vi "Set Isolated Crop Mode.vi"(6 "hbin":i32, 7 "vbin":i32, 9 "cropwidth":i32, 10 "cropheight":i32, 11 "active":i32) -> (3 "function return":u32)   [LabVIEW 2018, in "AndorSDK.lvlib"]
doc: "EXPNETTYPE unsigned int WINAPI SetIsolatedCropMode(int active, int cropheight, int cropwidth, int vbin, int hbin);"
uses:
  AndorSDK.lvlib
  ATMCD32D.dll
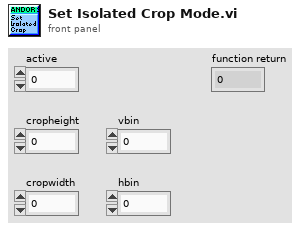
[diagram p1: front panel]
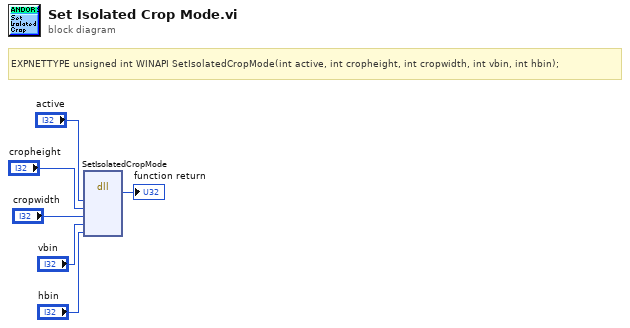
[diagram p0: block diagram]
diagram:
  # "EXPNETTYPE unsigned int WINAPI SetIsolatedCropMode(int active, int cropheight, int cropwidth, int vbin, int hbin);"
  n1 = dll-call lib="PTH2babs E\nPersönliches02 - Arbeit03-HiwijobsLabviewCodelibANDOR\tAndor SDK\nATMCD32D.*" fn="SetIsolatedCropMode"("active"="active", "cropheight"="cropheight", "cropwidth"="cropwidth", "vbin"="vbin", "hbin"="hbin") -> (→"function return":u32)  [unwired: 8 in, 2 out]
